vi "Check if Tab is Present.vi"(0 "vi in":refnum<vi>, 11 "error in":errorcluster) -> (4 "vi out":refnum<vi>, 8 "tab present?":bool, 15 "error out":errorcluster)   [LabVIEW 2021, in "Converter.lvlib"]
uses:
  Converter.lvlib
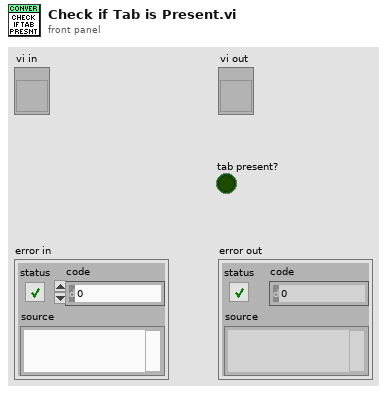
[diagram p1: front panel]
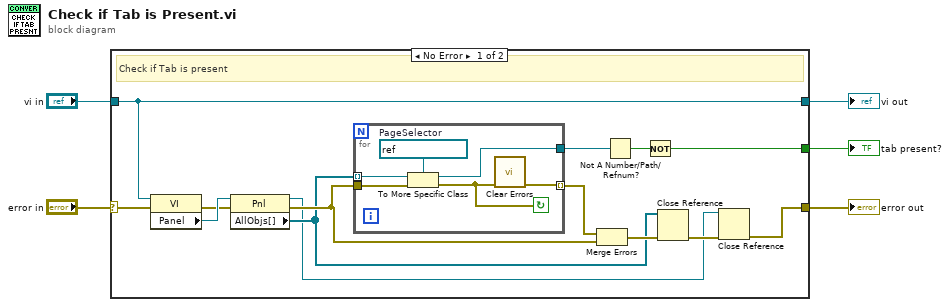
[diagram p0: block diagram]
diagram:
  n1 = case shown="No Error" "error in" {
    selector: "error in" -> [w18 w26]
    tunnel: [w10 w26] -> w5
    tunnel: [w15 w27] -> w4
    tunnel: "vi in" -> [w15 w27]
    tunnel: [w6 _] -> w1
    frame No Error {
      # "Check if Tab is present"
      n2 = property class="VI"(reference=w15, error in=w18) -> (error out=w17:errorcluster, "Panel"=w19:refnum<vi>)  [unwired: 1 out]
      n3 = property class="Pnl"(reference=w19, error in=w17) -> (reference out=w8:refnum<vi>, error out=w14:errorcluster, "AllObjs[]"=w11:refnum<vi>[])
      n4 = for {
        tunnel: w11 -> [w24] mode=indexing
        tunnel: w14 -> [w25]
        tunnel: [w20] -> w16 mode=indexing
        tunnel: [w21] -> w13
        stop <- w22 continue-if-true
        w23 = refnum<vi> refnum  # PageSelector
        n5 = To More Specific Class(target class=w23, reference=w24, error in=w25) -> (specific class reference=w21:refnum<vi>, error out=w22:errorcluster)
        n6 = call <vilib>:"Clear Errors.vi"("error in (no error)"=w22) -> ("error out"=w20:errorcluster)  [unwired: 5 in, 1 out]
      }
      n7 = Merge Errors(w16, w14) -> (w12:errorcluster)
      n8 = Not A Number/Path/Refnum?(number/path/refnum=w13) -> (NaN/Path/Refnum?=w7:bool)
      n9 = Not(x=w7) -> (.not. x?=w6:bool)
      n10 = Close Reference(reference=w11, error in (no error)=w12) -> (error out=w9:errorcluster)
      n11 = Close Reference(reference=w8, error in (no error)=w9) -> (error out=w10:errorcluster)
    }
    frame Error {
    }
  }
  "error out" <- w5
  "vi out" <- w4
  "tab present?" <- w1
